vi "addEmpProj.vi"(0 "Identifiant Projet":string, 1 "Identifiant Emp":string, 2 "OK Button":bool) -> ()   [LabVIEW 2023]
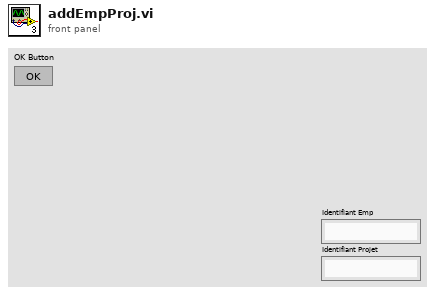
[diagram p1: front panel]
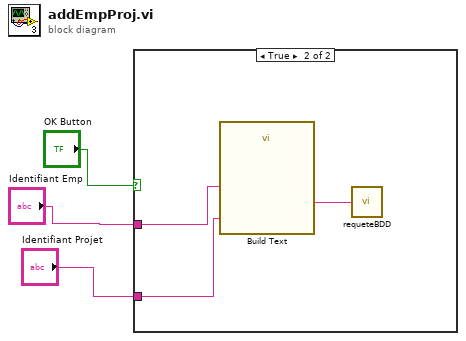
[diagram p0: block diagram]
diagram:
  n1 = case shown="True" "OK Button" {
    tunnel: "Identifiant Emp" -> [_ w6]
    tunnel: "Identifiant Projet" -> [_ w4]
    frame False {
    }
    frame True {
      n2 = call "Build Text"("id_emp"=w6, "id_projet"=w4) -> ("Result"=w5:string)  [unwired: 12 in, 1 out]
      n3 = call "requeteBDD.vi"("Requête Sql"=w5) -> ()  [unwired: 1 out]
    }
  }
